vi "GetWires.vi"(6 "error in":errorcluster, 9 "Diagram in":refnum<class "Diagram.lvclass">) -> (0 "error out":errorcluster, 3 "Diagram out":refnum<class "Diagram.lvclass">, 4 "wires":i32[](array[numeric]))   [LabVIEW 2014, in "Diagram.lvclass"]
uses:
  Diagram.lvclass
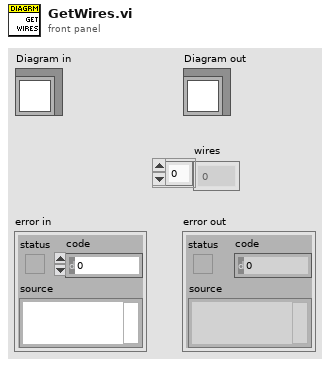
[diagram p1: front panel]
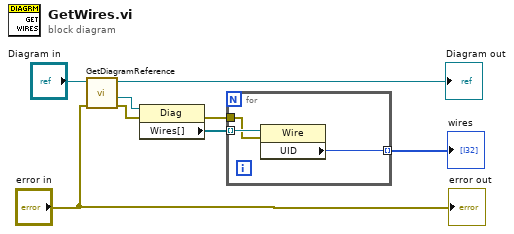
[diagram p0: block diagram]
diagram:
  n1 = call "GetDiagramReference.vi"("error in"="error in", "Diagram in"="Diagram in") -> ("error out"=w4:errorcluster, "reference out"=w5:refnum<vi>, "Diagram out"=→"Diagram out":refnum<class "Diagram.lvclass">)  [unwired: 5 in]
  n2 = property class="Diag"(reference=w5, error in=w4) -> (error out=w7:errorcluster, "Wires[]"=w8:refnum<vi>[])  [unwired: 1 out]
  n3 = for {
    tunnel: w8 -> [w11] mode=indexing
    tunnel: w7 -> [w10]
    tunnel: [w9] -> w1 mode=indexing
    n4 = property class="Wire"(reference=w11, error in=w10) -> ("UID"=w9:i32)  [unwired: 2 out]
  }
  "wires" <- w1
  "error out" <- "error in"
